vi "Read Append_.vi"(8 "error in (no error)":errorcluster, 11 "Report File in":refnum<class "Report File.lvclass">) -> (0 "error out":errorcluster, 2 "Append?":bool, 3 "Report File out":refnum<class "Report File.lvclass">)   [LabVIEW 2018, in "Report File.lvclass"]
uses:
  Report File.lvclass
  Report File.lvclass/Report File.ctl
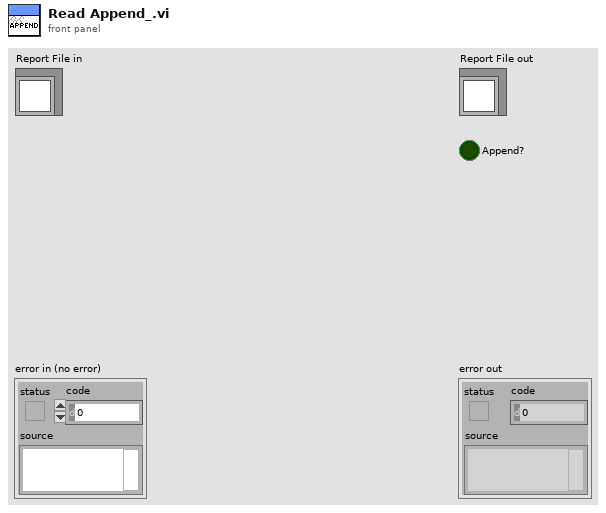
[diagram p1: front panel]
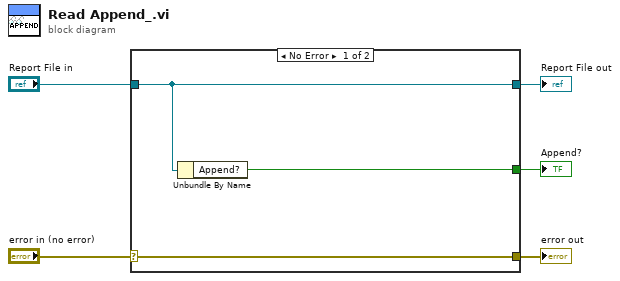
[diagram p0: block diagram]
diagram:
  n1 = case shown="No Error" "error in (no error)" {
    selector: "error in (no error)" -> [w8 w9]
    tunnel: [w8 w9] -> w4
    tunnel: [w7 w10] -> w2
    tunnel: "Report File in" -> [w7 w10]
    tunnel: [w6 _] -> w1
    frame No Error {
      n2 = Unbundle By Name(w7) -> ("Append?"=w6:bool)
    }
    frame Error {
    }
  }
  "error out" <- w4
  "Report File out" <- w2
  "Append?" <- w1
